vi "4Pi Focus Lock - 2D Gaussian - Fit Image U16.vi"(7 "Image In (U16)":u16[][](array[numeric]), 11 "Error In":errorcluster) -> (8 "Best Fit Params":T1, 15 "Error Out":errorcluster)   [LabVIEW 2016]
uses:
  Tools/2D Gaussian Fit/2D Gaussian - Type Defs/2D Gaussian - Best Fit Parameters.ctl
  <vilib>/gmath/NumericalOptimization/Nonlinear Curve Fit LM bound.vi
  <vilib>/gmath/NI_Gmath.lvlib
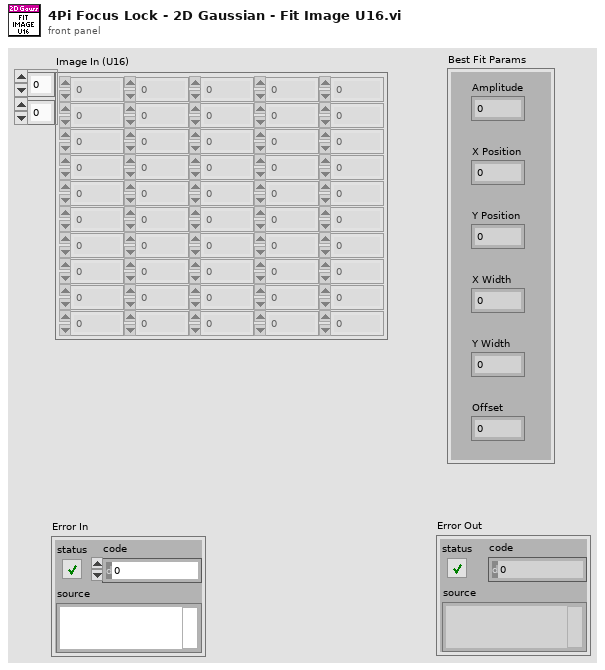
[diagram p1: front panel]
types:
  T1 = typedef "2D Gaussian - Best Fit Parameters.ctl" = cluster{"Amplitude":dbl, "X Position":dbl, "Y Position":dbl, "X Width":dbl, "Y Width":dbl, "Offset":dbl}
  T2 = cluster{"parameter minimum":dbl[], "parameter maximum":dbl[]}
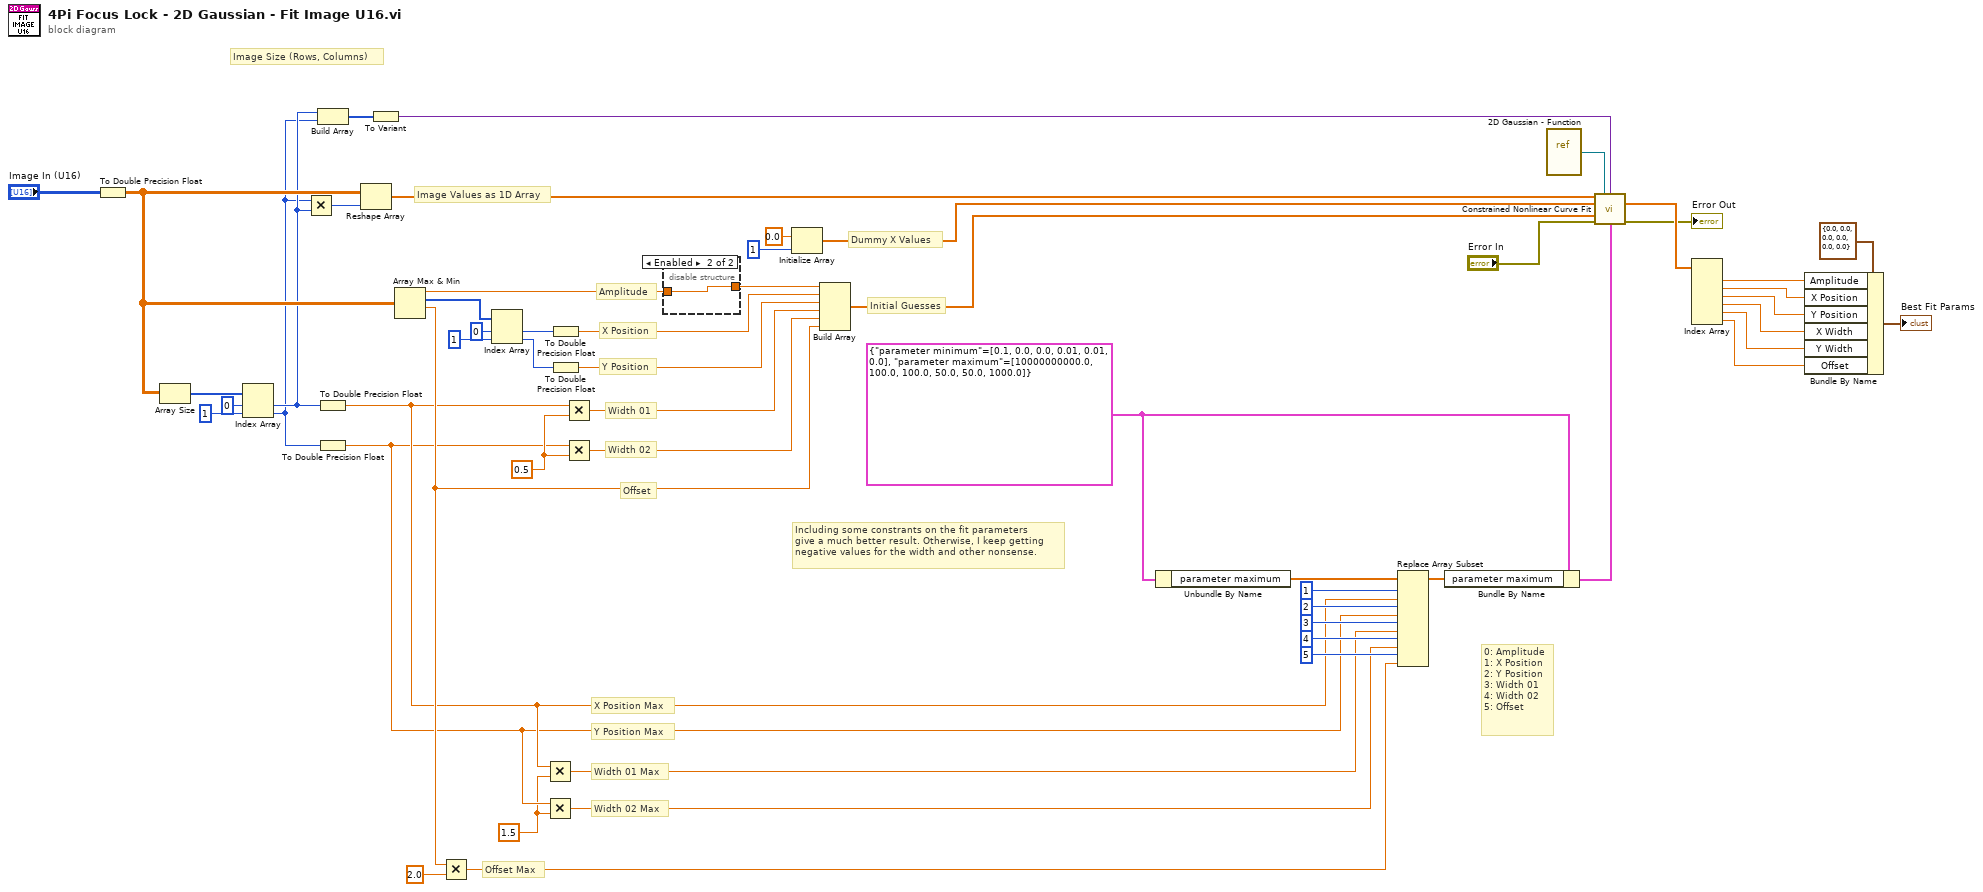
[diagram p0: block diagram]
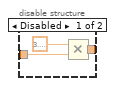
[diagram p2: hidden frame]
diagram:
  w3 = 1.5 ("y")
  w17 = T2 {"parameter minimum"=[0.1, 0.0, 0.0, 0.01, 0.01, 0.0], "parameter maximum"=[10000000000.0, 100.0, 100.0, 50.0, 50.0, 1000.0]} ("parameter bounds")
  w42 = 0.5
  # "Width 02 Max"
  # "Width 01 Max"
  # "Y Position Max"
  # "X Position Max"
  # "Offset Max"
  # "0: Amplitude\n1: X Position\n2: Y Position\n3: Width 01\n4: Width 02\n5: Offset"
  # "Image Size (Rows, Columns)"
  # "Including some constrants on the fit parameters\ngive a much better result. Otherwise, I keep getting\nnegative values for the width and other nonsense."
  # "Dummy X Values"
  # "Image Values as 1D Array"
  # "Initial Guesses"
  # "Width 02"
  # "Width 01"
  # "Y Position"
  # "X Position"
  # "Offset"
  # "Amplitude"
  n1 = To Double Precision Float(number="Image In (U16)") -> (double precision float=w35:dbl[][])
  n2 = Array Size(array=w35) -> (size(s)=w43:i32[])
  n3 = Index Array(array=w43, index #1=0 ("index"), index #2=1 ("index")) -> (element #1=w33:i32, element #2=w32:i32)
  n4 = Multiply(x=w32, y=w33) -> (x*y=w38:i32)
  n5 = Build Array(w33, w32) -> (w31:i32[])
  n6 = To Double Precision Float(number=w33) -> (double precision float=w5:dbl)
  n7 = To Double Precision Float(number=w32) -> (double precision float=w4:dbl)
  n8 = Reshape Array(w35, w38) -> (w39:dbl[])
  n9 = To Variant(anything=w31) -> (Variant=w30:variant)
  n10 = Array Max & Min(array=w35) -> (max value=w54:dbl, max index (indices)=w52:i32[], min value=w19:dbl)  [unwired: 1 out]
  n11 = Multiply(x=w19, y=2.0) -> (x*y=w6:dbl)
  n12 = Index Array(array=w52, index #1=0 ("index"), index #2=1 ("index")) -> (element #1=w49:i32, element #2=w47:i32)
  n13 = Multiply(x=w5, y=w3) -> (x*y=w2:dbl)
  n14 = Multiply(x=w4, y=w3) -> (x*y=w1:dbl)
  n15 = To Double Precision Float(number=w49) -> (double precision float=w48:dbl)
  n16 = To Double Precision Float(number=w47) -> (double precision float=w46:dbl)
  n17 = Multiply(x=w5, y=w42) -> (x*y=w41:dbl)
  n18 = Multiply(x=w4, y=w42) -> (x*y=w40:dbl)
  n19 = disable-structure shown="Enabled" {
    disable-tunnel: w54 -> [w58 w60]
    disable-tunnel: [w57 w60] -> w53
    frame Disabled {
      n20 = Multiply(x=3.141592653589793, y=w58) -> (x*y=w57:dbl)
    }
    frame Enabled {
    }
  }
  n21 = Initialize Array(0.0 ("element"), 1 ("dimension size")) -> (w36:dbl[])
  n22 = Build Array(w53, w48, w46, w41, w40, w19) -> (w34:dbl[])
  n23 = Unbundle By Name(w17) -> ("parameter maximum"=w16:dbl[])
  n24 = Replace Array Subset(array=w16, new element #1=w5, index #1=1 ("index"), new element #2=w4, index #2=2 ("index"), new element #3=w2, index #3=3 ("index"), new element #4=w1, index #4=4 ("index"), new element #5=w6, index #5=5 ("index")) -> (w15:dbl[])
  n25 = Bundle By Name(cluster=w17, "parameter maximum"=w15) -> (w14:T2)
  n26 = vi-ref "2D Gaussian - Function.vi"() -> (w56:refnum<vi>)
  n27 = call-poly <vilib>:"Constrained Nonlinear Curve Fit.vi"("Y"=w39, "f(x,a)"=w56, "data"=w30, "X"=w36, "initial parameters"=w34, "error in (no error)"="Error In", "parameter bounds"=w14) -> ("best fit parameters"=w28:dbl[], "error out"=→"Error Out":errorcluster)  [unwired: 3 in, 4 out]
  n28 = Index Array(array=w28) -> (element #1=w27:dbl, element #2=w26:dbl, element #3=w25:dbl, element #4=w24:dbl, element #5=w23:dbl, element #6=w22:dbl)  [unwired: 6 in]
  n29 = Bundle By Name(cluster=T1 {"Amplitude"=0.0, "X Position"=0.0, "Y Position"=0.0, "X Width"=0.0, "Y Width"=0.0, "Offset"=0.0} ("Best Fit Parameters"), "Amplitude"=w27, "X Position"=w26, "Y Position"=w25, "X Width"=w24, "Y Width"=w23, "Offset"=w22) -> (→"Best Fit Params":T1)
